vi "AxisNameTonumber.vi"(10 "Channel":string, 11 "Tapedrive_ESP301 in":refnum<class "Tapedrive_ESP301.lvclass">) -> (2 "Axis No.":i16, 3 "Tapedrive_ESP301 out":refnum<class "Tapedrive_ESP301.lvclass">)   [LabVIEW 2013, in "Tapedrive_ESP301.lvclass"]
uses:
  Tapedrive_ESP301.lvclass
  Tapedrive_ESP301.lvclass/Tapedrive_ESP301.ctl
panel:
  out "appended array":i16[](array[numeric])
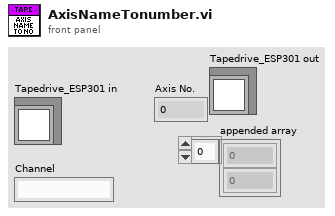
[diagram p1: front panel]
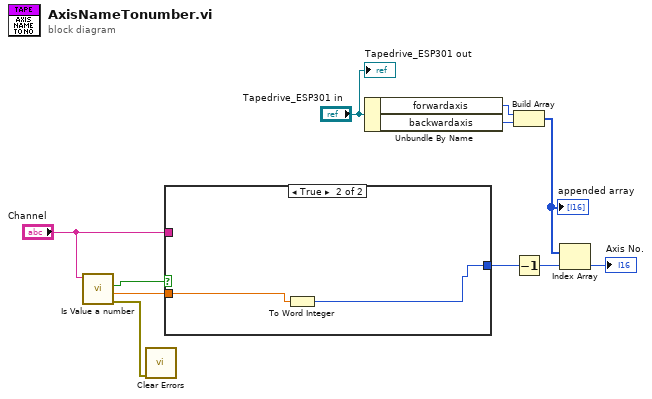
[diagram p0: block diagram]
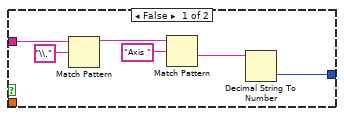
[diagram p2: hidden frame]
diagram:
  n1 = call "Is Value a number.vi"("value String"="Channel") -> ("user error out"=w1:errorcluster, "number"=w2:dbl, "a number"=w3:bool)  [unwired: 7 in, 1 out]
  n2 = call <vilib>:"Clear Errors.vi"("error in (no error)"=w1) -> ()  [unwired: 6 in, 1 out]
  n3 = case shown="True" w3 {
    tunnel: [w17 w18] -> w7
    tunnel: "Channel" -> [w12 _]
    tunnel: w2 -> [_ w19]
    frame False {
      n4 = Match Pattern(string=w12, regular expression="\\.") -> (before substring=w15:string)  [unwired: 1 in, 3 out]
      n5 = Match Pattern(string=w15, regular expression="Axis ") -> (after substring=w13:string)  [unwired: 1 in, 3 out]
      n6 = Decimal String To Number(string=w13) -> (number=w17:i32)  [unwired: 2 in, 1 out]
    }
    frame True {
      n7 = To Word Integer(number=w19) -> (16bit integer=w18:i16)
    }
  }
  n8 = Unbundle By Name("Tapedrive_ESP301 in") -> ("forwardaxis"=w5:i16, "backwardaxis"=w6:i16)
  n9 = Build Array(w5, w6) -> (w9:i16[])
  "appended array" <- w9
  n10 = Decrement(x=w7) -> (x-1=w8:i32)
  n11 = Index Array(array=w9, index=w8) -> (element=→"Axis No.":i16)
  "Tapedrive_ESP301 out" <- "Tapedrive_ESP301 in"
